vi "RM.findServerByGUID.vi"(8 "error in":errorcluster, 10 "serverGUID":string, 11 "Item Ref in":T1 format="%.0x") -> (0 "error out":errorcluster, 1 "found?":bool, 2 "serverInfo":T2 {"cd node ref" format="%.0x"}, 3 "Item Ref out":T1 format="%.0x")   [LabVIEW 2016, in "FPGA Resource Manager.lvlib"]
uses:
  FPGA Resource Manager.lvlib
  RM.serverInfo.ctl
  <vilib>/NI Veristand/Custom Device API/Custom Device Item Ref.ctl
  <vilib>/NI Veristand/Custom Device API/Custom Device API.lvlib
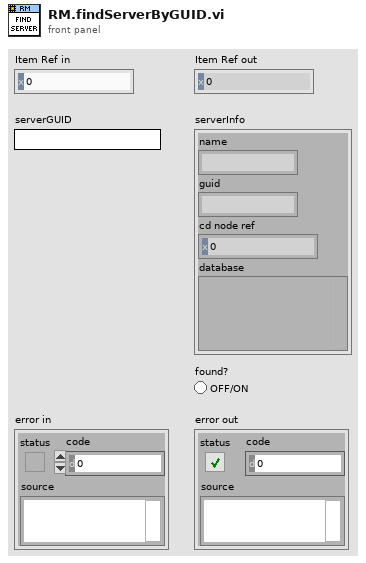
[diagram p1: front panel]
types:
  T1 = typedef "Custom Device API.lvlib/Custom Device Item Ref.ctl" = u64
  T2 = typedef "FPGA Resource Manager.lvlib/RM.serverInfo.ctl" = cluster{"name":string, "guid":string, "cd node ref":T1, "database":variant}
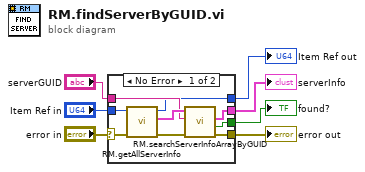
[diagram p0: block diagram]
diagram:
  n1 = case shown="No Error" "error in" {
    selector: "error in" -> [w12 w17]
    tunnel: "serverGUID" -> [w15 _]
    tunnel: [w14 _] -> w2
    tunnel: [w13 _] -> w1
    tunnel: "Item Ref in" -> [w11 w18]
    tunnel: [w8 w17] -> w4
    tunnel: [w10 w18] -> w3
    frame No Error {
      n2 = call "RM.getAllServerInfo.vi"("error in"=w12, "Item Ref in"=w11) -> ("error out"=w9:errorcluster, "ServerInfo Array"=w16:T2[], "Item Ref out"=w10:T1)  [unwired: 7 in]
      n3 = call "RM.searchServerInfoArrayByGUID.vi"("error in (no error)"=w9, "selected deviceGUID"=w15, "serverInfo array in"=w16) -> ("error out"=w8:errorcluster, "found?"=w13:bool, "serverInfo"=w14:T2)  [unwired: 5 in, 1 out]
    }
    frame Error {
    }
  }
  "found?" <- w1
  "serverInfo" <- w2
  "error out" <- w4
  "Item Ref out" <- w3
